vi "Climb Solenoid.vi"(10 "Value":T4, 11 "Enum":enum16{"Start", "Run", "End"}(ring)=enum."Run") -> ()   [LabVIEW 2012]
uses:
  <vilib>/Rock Robotics/WPI/Solenoid/WPI_SolenoidValue.ctl
  <vilib>/Rock Robotics/WPI/Solenoid/WPI_SolenoidChannel.ctl
  <vilib>/Rock Robotics/SystemInterfaces/Typedef/FPGA_TypedefSolenoidModule.ctl
  <vilib>/Rock Robotics/WPI/Solenoid/WPI_SolenoidOpenSingle.vi
  <vilib>/Rock Robotics/WPI/Solenoid/WPI_SolenoidSetEnum.vi
panel:
  in  "Solenoid Module 1":T3={"Shoot FWD"=enum."Solenoid 1", "Shoot REV"=enum."Solenoid 2", "Climber"=enum."Solenoid 3", "Climber"=enum."Solenoid 4", "Arm Lock"=enum."Solenoid 5", "Unassigned"=enum."Solenoid 6", "Color"=enum."Solenoid 7", "Unassigned"=enum."Solenoid 8", "Module"=enum."Solenoid Module 1"}
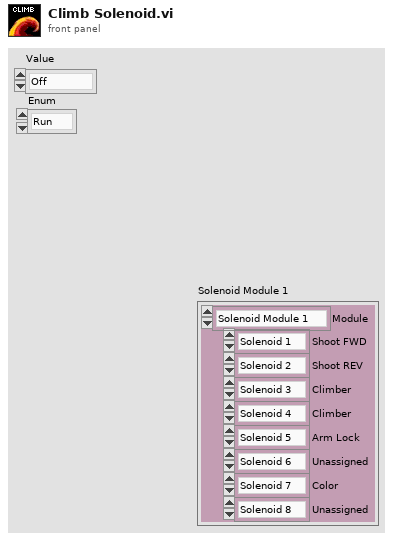
[diagram p1: front panel]
types:
  T1 = typedef "WPI_SolenoidChannel.ctl" = enum8{"Solenoid 1", "Solenoid 2", "Solenoid 3", "Solenoid 4", "Solenoid 5", "Solenoid 6", "Solenoid 7", "Solenoid 8", "Invalid"}
  T2 = typedef "FPGA_TypedefSolenoidModule.ctl" = enum16{"Solenoid Module 1", "Solenoid Module 2"}
  T3 = cluster{"Shoot FWD":T1, "Shoot REV":T1, "Climber":T1, "Climber":T1, "Arm Lock":T1, "Unassigned":T1, "Color":T1, "Unassigned":T1, "Module":T2}
  T4 = typedef "WPI_SolenoidValue.ctl" = enum16{"Off", "On", "Forward", "Reverse"}
  T5 = typedef "WPI_SolenoidDevRef.ctl" = cluster{"DevStatus":errorcluster, "Solenoid Module":T2, "Forward Solenoid Channel":T1, "Reverse Solenoid Channel":T1}
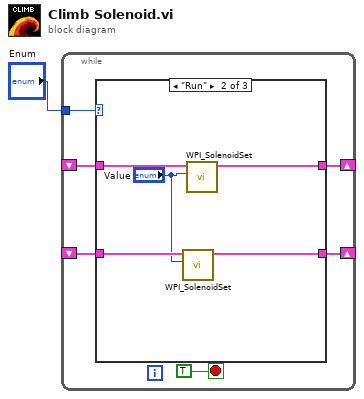
[diagram p0: block diagram]
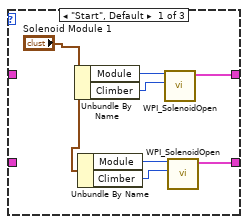
[diagram p2: hidden frame]
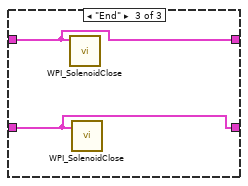
[diagram p3: hidden frame]
diagram:
  n1 = while {
    tunnel: "Enum" -> [w6]
    shift-right: [w5] -> _
    shift-left: _ -> [w4]
    shift-right: [w3] -> _
    shift-left: _ -> [w2]
    stop <- TRUE stop-if-true
    n2 = case shown="\"Run\"" w6 {
      tunnel: [w12 w18 w21] -> w5
      tunnel: w4 -> [_ w19 w21]
      tunnel: [w8 w16 w20] -> w3
      tunnel: w2 -> [_ w17 w20]
      frame "Start", Default {
        n3 = Unbundle By Name("Solenoid Module 1") -> ("Module"=w14:T2, "Climber"=w13:T1)
        n4 = Unbundle By Name("Solenoid Module 1") -> ("Module"=w11:T2, "Climber"=w10:T1)
        n5 = call-poly <vilib>:"WPI_SolenoidOpen.vi"("Solenoid Channel"=w13, "Solenoid Module (Module 1)"=w14) -> ("SolenoidDevRef"=w12:T5)  [unwired: 8 in, 1 out]
        n6 = call-poly <vilib>:"WPI_SolenoidOpen.vi"("Solenoid Channel"=w10, "Solenoid Module (Module 1)"=w11) -> ("SolenoidDevRef"=w8:T5)  [unwired: 8 in, 1 out]
      }
      frame "Run" {
        n7 = call-poly <vilib>:"WPI_SolenoidSet.vi"("Value"="Value", "SolenoidDevRef"=w17) -> ("SolenoidDevRef"=w16:T5)  [unwired: 8 in, 1 out]
        n8 = call-poly <vilib>:"WPI_SolenoidSet.vi"("Value"="Value", "SolenoidDevRef"=w19) -> ("SolenoidDevRef"=w18:T5)  [unwired: 8 in, 1 out]
      }
      frame "End" {
        n9 = call <vilib>:"WPI_SolenoidClose.vi"("SolenoidDevRef"=w21) -> ()  [unwired: 10 in, 1 out]
        n10 = call <vilib>:"WPI_SolenoidClose.vi"("SolenoidDevRef"=w20) -> ()  [unwired: 10 in, 1 out]
      }
    }
  }
